vi "main-aq-program.vi"() -> ()   [LabVIEW 2015]
uses:
  <vilib>/userdefined/High Color/IMAQdx.ctl
  globals.vi
  <vilib>/vision/driver/NI_Vision_Acquisition_Software.lvlib
  <resource>/objmgr/imaqdx.rc
panel:
  in  "Save image":bool
  in  "Name":string
  in  "Path":path
  out "Image 2":T1(plugin-control)
  out "Image":T1(plugin-control)
  in  "Camera-right":T2="cam4"
  in  "Exposure time left":dbl=10000.0
  in  "Stop Button":bool
  in  "Camera-left":T2="cam4"
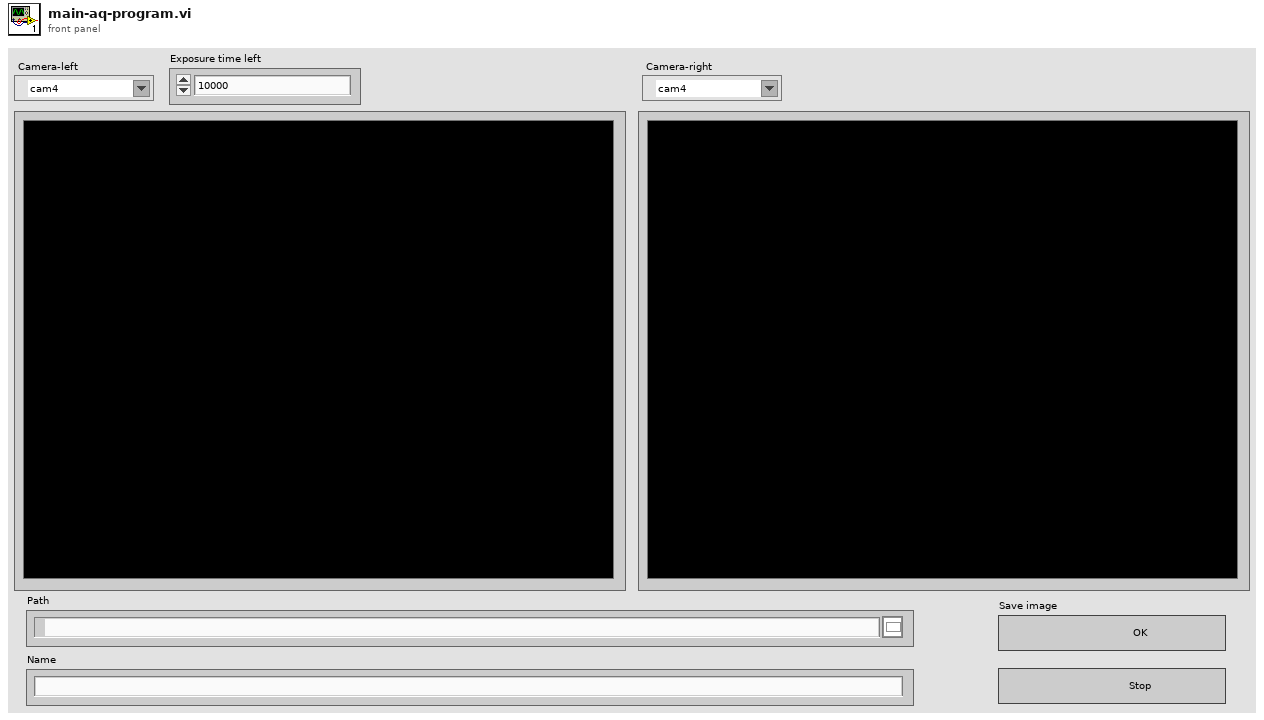
[diagram p1: front panel]
types:
  T1 = typedef "IMAQ Image.ctl" = refnum<image>
  T2 = typedef "IMAQdx.ctl" = refnum<k21>
  T3 = typedef "Image Type" = u32
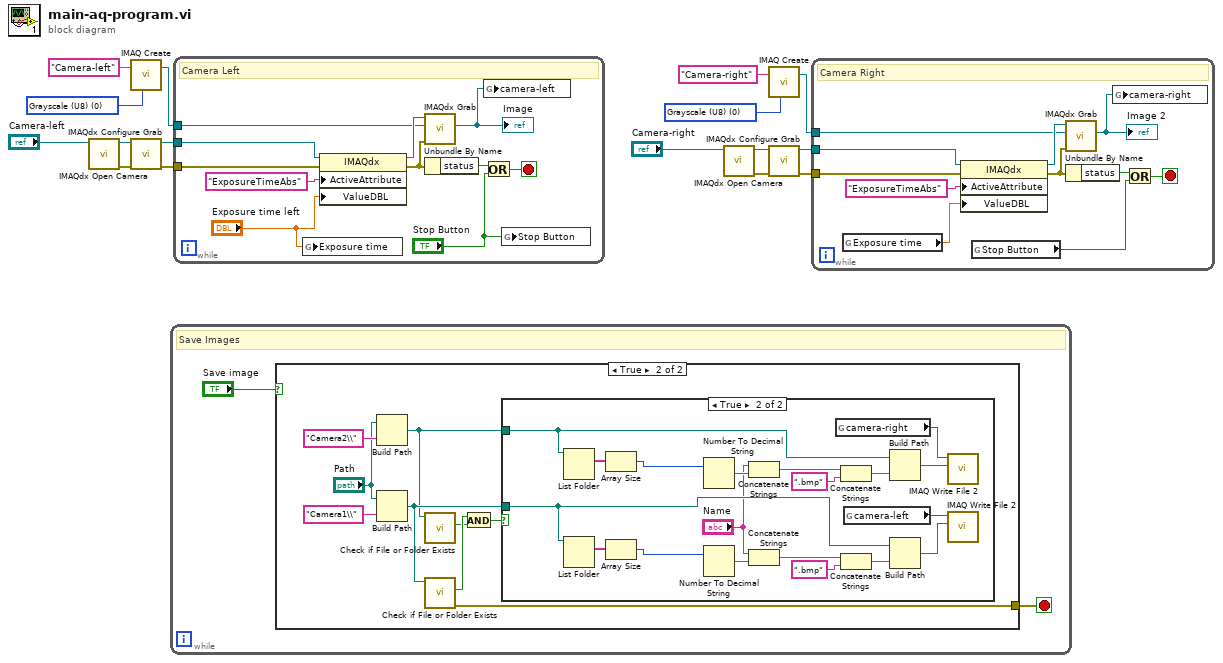
[diagram p0: block diagram]
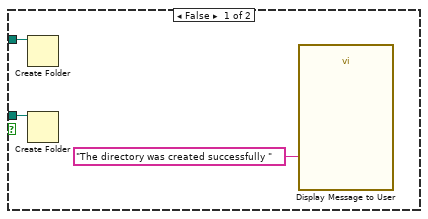
[diagram p3: hidden frame]
diagram:
  w10 = T3 0 items=["Grayscale (U8)", "Grayscale (I16)", "Grayscale (SGL)", "Complex (CSG)", "RGB (U32)", "HSL (U32)", "RGB (U64)"] ("Image Type")
  w16 = T3 0 items=["Grayscale (U8)", "Grayscale (I16)", "Grayscale (SGL)", "Complex (CSG)", "RGB (U32)", "HSL (U32)", "RGB (U64)"] ("Image Type")
  n1 = call <vilib>:"IMAQdx Open Camera.vi"("Session In"="Camera-left") -> ("error out"=w3:errorcluster, "Session Out"=w4:T2)  [unwired: 2 in, 7 out]
  n2 = call "IMAQ Create"("Image Name"="Camera-left", "Image Type"=w16) -> ("New Image"=w11:T1)  [unwired: 2 in, 2 out]
  n3 = call <vilib>:"IMAQdx Configure Grab.vi"("error in"=w3, "Session In"=w4) -> ("error out"=w12:errorcluster, "Session Out"=w13:T2)  [unwired: 8 out]
  n4 = while {
    stop <- w18 stop-if-true
    # "Save Images"
    n5 = case shown="True" "Save image" {
      tunnel: [_ w25] -> w18
      frame False {
      }
      frame True {
        n6 = Build Path(base path="Path", name or relative path="Camera2\\") -> (appended path=w20:path)
        n7 = Build Path(base path="Path", name or relative path="Camera1\\") -> (appended path=w26:path)
        n8 = call <vilib>:"Check if File or Folder Exists.vi"("path"=w20) -> ("file or folder exists?"=w22:bool)  [unwired: 8 in, 2 out]
        n9 = call <vilib>:"Check if File or Folder Exists.vi"("path"=w26) -> ("error out"=w25:errorcluster, "file or folder exists?"=w23:bool)  [unwired: 8 in, 1 out]
        n10 = And(x=w23, y=w22) -> (x .and. y?=w21:bool)
        n11 = case shown="True" w21 {
          tunnel: w26 -> [w30 w38]
          tunnel: w20 -> [w29 w39]
          frame False {
            n12 = Create Folder(path (use dialog)=w29) -> ()  [unwired: 2 in, 3 out]
            n13 = Create Folder(path (use dialog)=w30) -> ()  [unwired: 2 in, 3 out]
            n14 = call "Display Message to User"("Message"="The directory was created successfully ") -> ()  [unwired: 9 in, 2 out]
          }
          frame True {
            n15 = List Folder(path=w39) -> (filenames=w44:string[])  [unwired: 3 in, 3 out]
            n16 = List Folder(path=w38) -> (filenames=w49:string[])  [unwired: 3 in, 3 out]
            n17 = Array Size(array=w44) -> (size(s)=w32:i32)
            n18 = Array Size(array=w49) -> (size(s)=w31:i32)
            n19 = Number To Decimal String(number=w32) -> (decimal integer string=w43:string)  [unwired: 1 in]
            n20 = Number To Decimal String(number=w31) -> (decimal integer string=w48:string)  [unwired: 1 in]
            n21 = Concatenate Strings("Name", w43) -> (w42:string)
            n22 = Concatenate Strings("Name", w48) -> (w47:string)
            n23 = global read "globals.vi" "camera-right"() -> (w35:T1)
            n24 = Concatenate Strings(w42, ".bmp") -> (w40:string)
            n25 = Concatenate Strings(w47, ".bmp") -> (w45:string)
            n26 = global read "globals.vi" "camera-left"() -> (w33:T1)
            n27 = Build Path(base path=w39, name or relative path=w40) -> (appended path=w36:path)
            n28 = Build Path(base path=w38, name or relative path=w45) -> (appended path=w34:path)
            n29 = call-poly "IMAQ Write File 2"("File Path"=w36, "Image"=w35) -> ()  [unwired: 8 in, 2 out]
            n30 = call-poly "IMAQ Write File 2"("File Path"=w34, "Image"=w33) -> ()  [unwired: 8 in, 2 out]
          }
        }
      }
    }
  }
  n31 = while {
    tunnel: w13 -> [w55]
    tunnel: w12 -> [w54]
    tunnel: w11 -> [w53]
    stop <- w57 stop-if-true
    # "Camera Left"
    n32 = global write "globals.vi" "Exposure time"("Exposure time left") -> ()
    n33 = property on="Property Node left" class="IMAQdx"(reference=w55, error in=w54, "ActiveAttribute"="ExposureTimeAbs" ("String"), "ValueDBL"="Exposure time left") -> (reference out=w59:T2, error out=w56:errorcluster)
    n34 = call <vilib>:"IMAQdx Grab.vi"("error in"=w56, "Image In"=w53, "Session In"=w59) -> ("Image Out"=w50:T1)  [unwired: 1 in, 7 out]
    "Image" <- w50
    n35 = Unbundle By Name(w56) -> ("status"=w58:bool)
    n36 = global write "globals.vi" "camera-left"(w50) -> ()
    n37 = Or(x=w58, y="Stop Button") -> (x .or. y?=w57:bool)
    n38 = global write "globals.vi" "Stop Button"("Stop Button") -> ()
  }
  n39 = call <vilib>:"IMAQdx Open Camera.vi"("Session In"="Camera-right") -> ("error out"=w1:errorcluster, "Session Out"=w2:T2)  [unwired: 2 in, 7 out]
  n40 = call "IMAQ Create"("Image Name"="Camera-right", "Image Type"=w10) -> ("New Image"=w5:T1)  [unwired: 2 in, 2 out]
  n41 = call <vilib>:"IMAQdx Configure Grab.vi"("error in"=w1, "Session In"=w2) -> ("error out"=w6:errorcluster, "Session Out"=w7:T2)  [unwired: 8 out]
  n42 = while {
    tunnel: w7 -> [w66]
    tunnel: w6 -> [w65]
    tunnel: w5 -> [w64]
    stop <- w68 stop-if-true
    # "Camera Right"
    n43 = global read "globals.vi" "Exposure time"() -> (w62:dbl)
    n44 = property on="Property Node left" class="IMAQdx"(reference=w66, error in=w65, "ActiveAttribute"="ExposureTimeAbs" ("String"), "ValueDBL"=w62) -> (reference out=w70:T2, error out=w67:errorcluster)
    n45 = global read "globals.vi" "Stop Button"() -> (w63:bool)
    n46 = call <vilib>:"IMAQdx Grab.vi"("error in"=w67, "Image In"=w64, "Session In"=w70) -> ("Image Out"=w61:T1)  [unwired: 1 in, 7 out]
    "Image 2" <- w61
    n47 = Unbundle By Name(w67) -> ("status"=w69:bool)
    n48 = global write "globals.vi" "camera-right"(w61) -> ()
    n49 = Or(x=w69, y=w63) -> (x .or. y?=w68:bool)
  }
